vi "EPICS scan.vi"() -> ()   [LabVIEW 2018]
uses:
  Motor-Scan setup.ctl
  <userlib>/caLab/Private/Put_DBL-1D_PV-1D.vi
  <userlib>/caLab/Private/Put_DBL_PV.vi
panel:
  out "Scan Inner Iterations":i32
  out "Scan Outer Iterations":i32
  out "Scan loop iterations":i32
  out "Command Loop iterations":i32
  in  "Scan Parameters":cluster{"Inner motor":T1, "Outer Motor":T1}={"Inner motor"={"Motor PV"="c3lm:aero:c0:m1", "Start Position"=-80.0, "End Position"=0.0, "Step Size"=20.0}, "Outer Motor"={"Motor PV"="c3lm:aero:c1:m1", "Start Position"=0.0, "End Position"=300.0, "Step Size"=30.0}}
  in  "Exposure Time (ms)":dbl=250.0
  out "Monitor Loop iterations":i32=694
  out "Waveform Chart":T2(graph)={"[0]"=0.0, "[1]"=200.0, "[2]"=0.0, "[3]"=0.0, "[4]"=0.0, "[5]"=0.0, "[6]"=0.0, "[7]"=0.0, "[8]"=0.0}
  in  "Monitor Frequency (Hz)":dbl=10.0
  in  "Start Scan":bool
  in  "Stop Program":bool
  in  "Stop Scan":bool
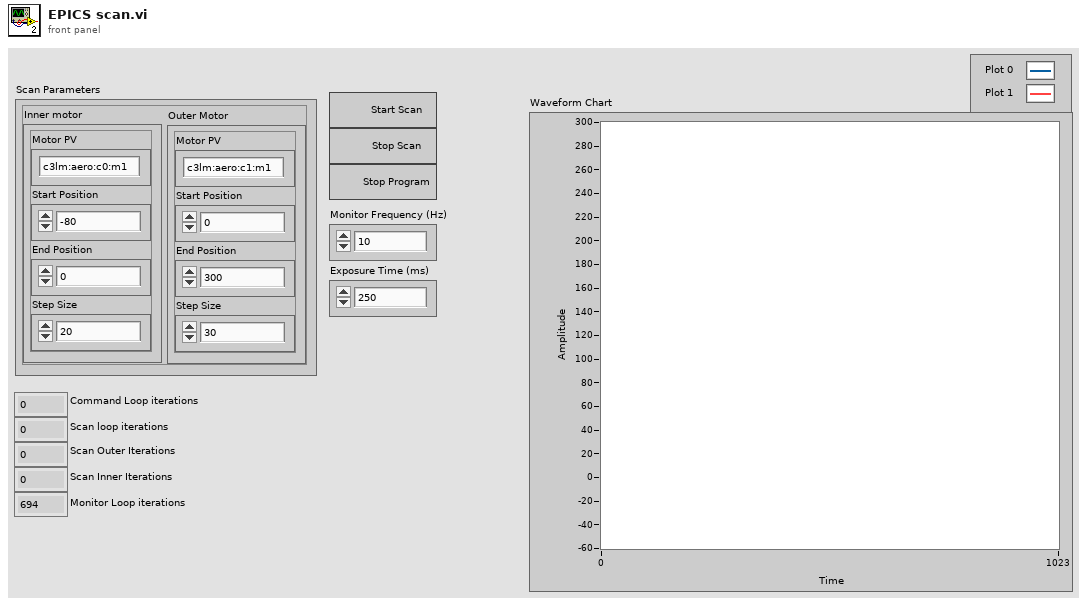
[diagram p1: front panel]
types:
  T1 = typedef "Motor-Scan setup.ctl" = cluster{"Motor PV":string, "Start Position":dbl, "End Position":dbl, "Step Size":dbl}
  T2 = cluster{"[0]":dbl, "[1]":dbl, "[2]":dbl, "[3]":dbl, "[4]":dbl, "[5]":dbl, "[6]":dbl, "[7]":dbl, "[8]":dbl}
  T3 = cluster{"Array out[0]":dbl, "Array out[1]":dbl, "Array out[2]":dbl, "Array out[3]":dbl, "Array out[4]":dbl, "Array out[5]":dbl, "Array out[6]":dbl, "Array out[7]":dbl, "Array out[8]":dbl}
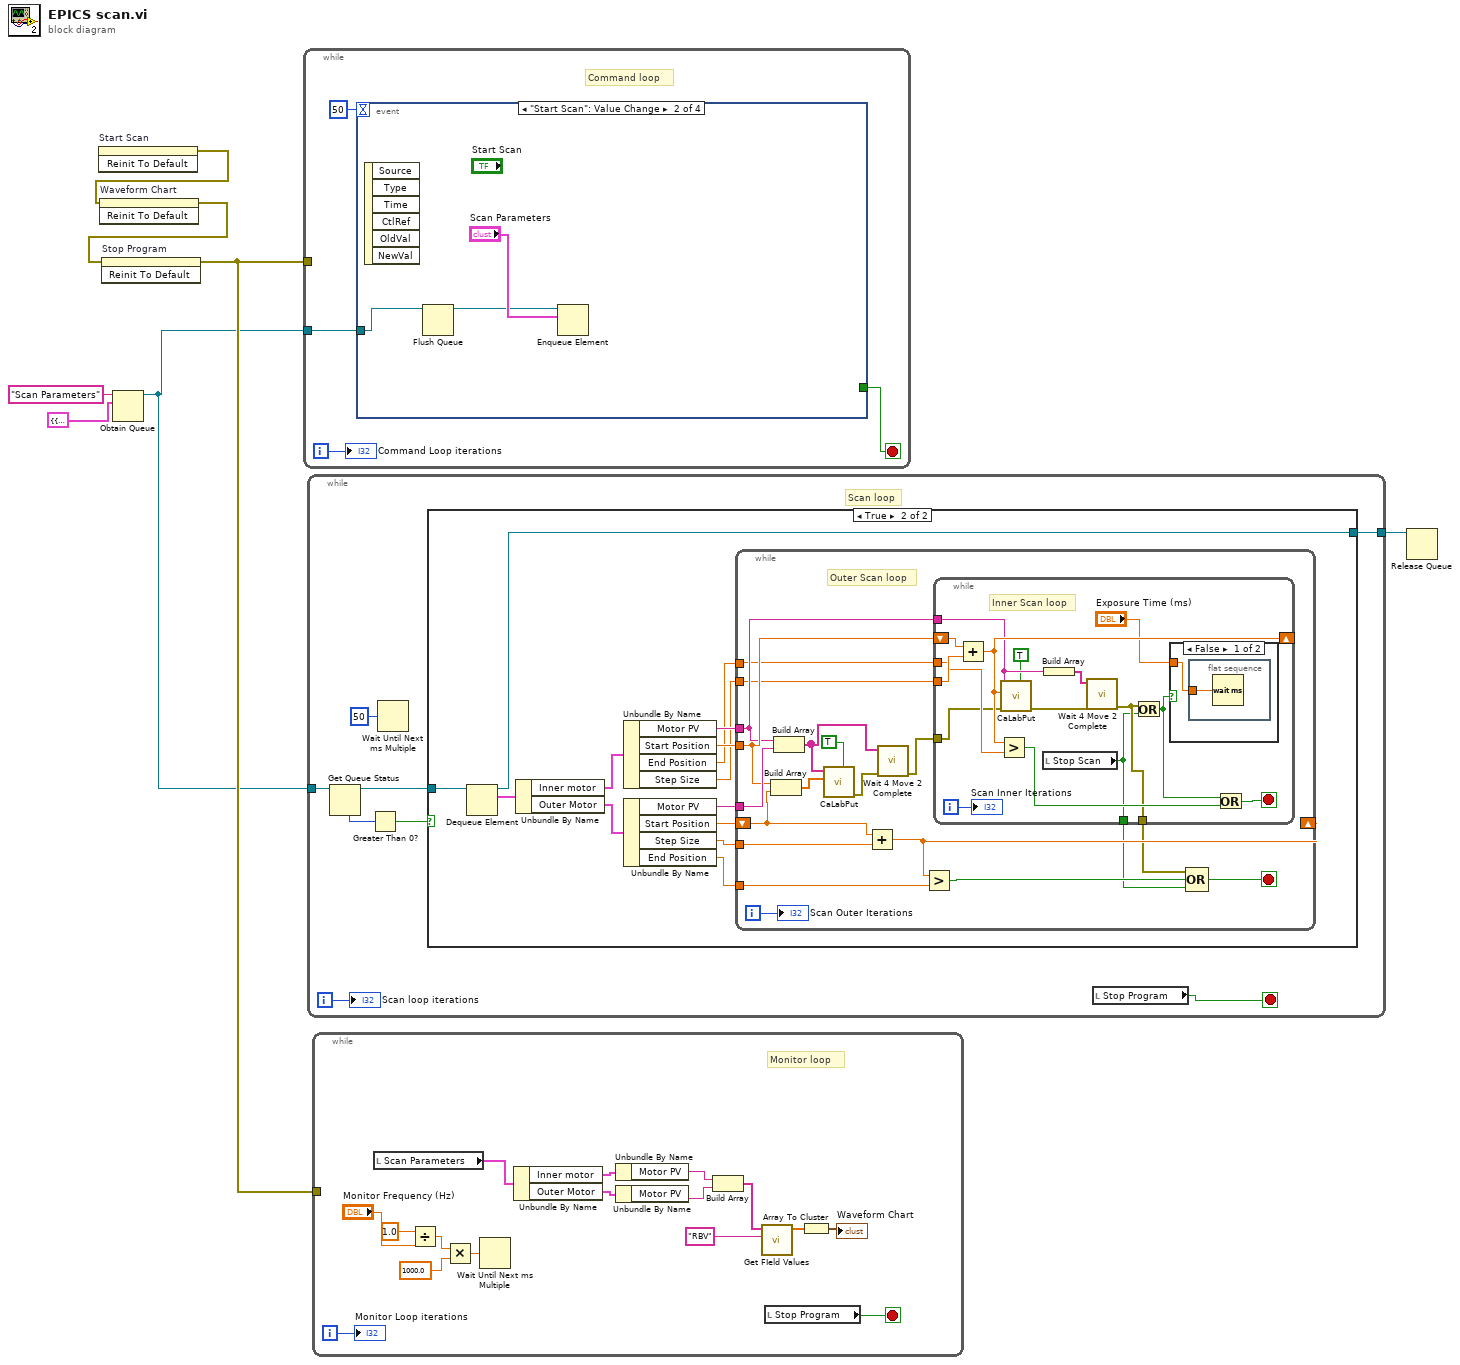
[diagram p0: block diagram]
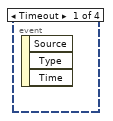
[diagram p4: hidden frame]
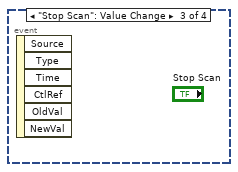
[diagram p5: hidden frame]
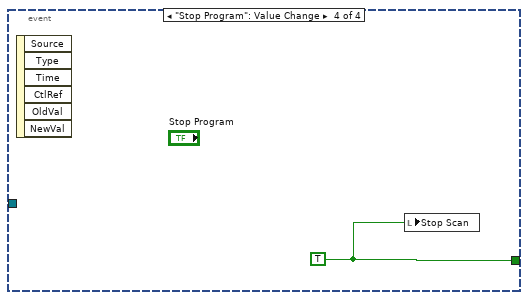
[diagram p6: hidden frame]
diagram:
  n1 = invoke on="Start Scan" class="Bool" method="Reinit To Default"() -> (error out=w6:errorcluster)  [unwired: 3 in, 2 out]
  n2 = invoke on="Waveform Chart" class="WFChart (strict)" method="Reinit To Default"(error in=w6) -> (error out=w7:errorcluster)  [unwired: 2 in, 2 out]
  n3 = invoke on="Stop Program" class="Bool (strict)" method="Reinit To Default"(error in=w7) -> (error out=w5:errorcluster)  [unwired: 2 in, 2 out]
  n4 = Obtain Queue(name (unnamed)="Scan Parameters", element data type=cluster{"Inner motor":T1, "Outer Motor":T1} {"Inner motor"={"Motor PV"="c3lm:aero:c0:m1", "Start Position"=0.0, "End Position"=-80.0, "Step Size"=20.0}, "Outer Motor"={"Motor PV"="c3lm:aero:c1:m1", "Start Position"=0.0, "End Position"=300.0, "Step Size"=30.0}} ("Scan Parameters 2")) -> (queue out=w2:refnum<queue>)  [unwired: 3 in, 2 out]
  n5 = while {
    tunnel: w5 -> [_]
    tunnel: w2 -> [w8]
    i -> [w9]
    stop <- w11 stop-if-true
    # "Command loop"
    n6 = event shown="[1] \"Start Scan\": Value Change" {
      selector: _ -> [_ _ _ _]
      dyn-events: _ -> [_ _ _ _]
      timeout: 50 -> [_ _ _ _]
      tunnel: [_ _ _ w15] -> w11
      tunnel: w8 -> [_ w14 _ _]
      event Timeout {
        n7 = event-data() -> ()  [unwired: 1 in, 3 out]
      }
      event "Start Scan": Value Change {
        n8 = event-data() -> ()  [unwired: 1 in, 6 out]
        n9 = Flush Queue(queue=w14) -> (queue out=w12:refnum<queue>)  [unwired: 1 in, 2 out]
        n10 = Enqueue Element(queue=w12, element="Scan Parameters") -> ()  [unwired: 2 in, 3 out]
      }
      event "Stop Scan": Value Change {
        n11 = event-data() -> ()  [unwired: 1 in, 6 out]
      }
      event "Stop Program": Value Change {
        w15 = TRUE
        n12 = event-data() -> ()  [unwired: 1 in, 6 out]
        n13 = local write "Stop Scan"(w15) -> ()
      }
    }
    "Command Loop iterations" <- w9
  }
  n14 = while {
    tunnel: w2 -> [w21]
    tunnel: [w17] -> w1
    i -> [w22]
    stop <- w23 stop-if-true
    # "Scan loop"
    n15 = Get Queue Status(queue=w21) -> (queue out=w18:refnum<queue>, # elements in queue=w20:i32)  [unwired: 2 in, 6 out]
    n16 = Greater Than 0?(x=w20) -> (x > 0?=w19:bool)
    n17 = Wait Until Next ms Multiple(millisecond multiple=u32 50 ("milliseconds to wait")) -> ()  [unwired: 1 out]
    n18 = case shown="True" w19 {
      tunnel: w18 -> [w24 w37]
      tunnel: [w24 w33] -> w17
      frame False {
      }
      frame True {
        n19 = Dequeue Element(queue=w37) -> (queue out=w33:refnum<queue>, element=w36:cluster{"Inner motor":T1, "Outer Motor":T1})  [unwired: 2 in, 2 out]
        n20 = Unbundle By Name(w36) -> ("Inner motor"=w35:T1, "Outer Motor"=w34:T1)
        n21 = Unbundle By Name(w35) -> ("Motor PV"=w30:string, "Start Position"=w32:dbl, "End Position"=w28:dbl, "Step Size"=w27:dbl)
        n22 = Unbundle By Name(w34) -> ("Motor PV"=w29:string, "Start Position"=w31:dbl, "Step Size"=w26:dbl, "End Position"=w25:dbl)
        n23 = while {
          shift-right: [w43] -> _
          shift-left: w31 -> [w45]
          tunnel: w30 -> [w49]
          tunnel: w29 -> [w56]
          tunnel: w32 -> [w50]
          tunnel: w28 -> [w48]
          tunnel: w27 -> [w47]
          tunnel: w26 -> [w46]
          tunnel: w25 -> [w44]
          i -> [w38]
          stop <- w42 stop-if-true
          # "Outer Scan loop"
          n24 = Build Array(w50, w45) -> (w55:dbl[])
          n25 = Build Array(w49, w56) -> (w52:string[])
          n26 = call-poly <userlib>:"CaLabPut.vi"("variable PV names (F)"=TRUE, "Values"=w55, "PV Names"=w52) -> ("Error out"=w53:errorcluster)  [unwired: 5 in, 3 out]
          n27 = Add(x=w45, y=w46) -> (x+y=w43:dbl)
          n28 = call "Wait 4 Move 2 Complete.vi"("error in (no error)"=w53, "Array"=w52) -> ("Error out"=w51:errorcluster)  [unwired: 9 in]
          n29 = Greater?(x=w43, y=w44) -> (0:w40:bool)
          n30 = while {
            tunnel: w51 -> [w65]
            tunnel: w49 -> [w67]
            shift-right: [w68] -> _
            shift-left: w50 -> [w71]
            tunnel: w48 -> [w69]
            tunnel: w47 -> [w70]
            tunnel: [w59] -> w41
            tunnel: [w58] -> w39
            i -> [w64]
            stop <- w61 stop-if-true
            # "Inner Scan loop"
            n31 = Add(x=w71, y=w70) -> (x+y=w68:dbl)
            n32 = Greater?(x=w68, y=w69) -> (0:w60:bool)
            n33 = call-poly <userlib>:"CaLabPut.vi"("variable PV names (F)"=TRUE, "Error in (no error)"=w65, "Value"=w68, "PV Name"=w67) -> ("Error out"=w72:errorcluster)  [unwired: 4 in, 3 out]
            n34 = local read "Stop Scan"() -> (w58:bool)
            n35 = Build Array(w67) -> (w66:string[])
            n36 = call "Wait 4 Move 2 Complete.vi"("error in (no error)"=w72, "Array"=w66) -> ("Error out"=w59:errorcluster)  [unwired: 9 in]
            n37 = Or(x=w59, y=w58) -> (x .or. y?=w57:bool)
            n38 = case shown="False" w57 {
              tunnel: "Exposure Time (ms)" -> [w73 _]
              frame False {
                n39 = flat-sequence {
                  tunnel: w73 -> [w74]
                  frame #0 {
                    n40 = Wait (ms)(milliseconds to wait=w74) -> ()  [unwired: 1 out]
                  }
                }
              }
              frame True {
              }
            }
            n41 = Or(x=w57, y=w60) -> (x .or. y?=w61:bool)
            "Scan Inner Iterations" <- w64
          }
          n42 = Compound Arithmetic op=OR(w41, w40, w39) -> (w42:bool)
          "Scan Outer Iterations" <- w38
        }
      }
    }
    n43 = local read "Stop Program"() -> (w23:bool)
    "Scan loop iterations" <- w22
  }
  n44 = while {
    tunnel: w5 -> [_]
    i -> [w81]
    stop <- w90 stop-if-true
    # "Monitor loop"
    n45 = local read "Scan Parameters"() -> (w76:cluster{"Inner motor":T1, "Outer Motor":T1})
    n46 = Divide(x=1.0, y="Monitor Frequency (Hz)") -> (x/y=w87:dbl)
    n47 = Multiply(x=w87, y=1000.0) -> (x*y=w84:dbl)
    n48 = Wait Until Next ms Multiple(millisecond multiple=w84) -> ()  [unwired: 1 out]
    n49 = Unbundle By Name(w76) -> ("Inner motor"=w80:T1, "Outer Motor"=w79:T1)
    n50 = Unbundle By Name(w80) -> ("Motor PV"=w77:string)
    n51 = Unbundle By Name(w79) -> ("Motor PV"=w78:string)
    n52 = Build Array(w77, w78) -> (w89:string[])
    n53 = call "Get FIeld Values.vi"("String"="RBV", "Array in"=w89) -> ("Array out"=w83:dbl[])  [unwired: 8 in, 1 out]
    n54 = local read "Stop Program"() -> (w90:bool)
    n55 = Array To Cluster(array=w83) -> (cluster=→"Waveform Chart":T3)
    "Monitor Loop iterations" <- w81
  }
  n56 = Release Queue(queue=w1) -> ()  [unwired: 2 in, 3 out]
